vi "Replacing The Heart - Lesson 8.vi"() -> ()   [LabVIEW 2023]
doc: "This lesson uses malleable VIs and LabVIEW classes without dynamic dispatching to solve the problem. The lesson introduces the concept of using malleable VIs to define an interface then allowing multiple LabVIEW classes to implement that interface."
uses:
  Person Information.ctl
  People Wrapper/People Wrapper.lvclass
  People Wrapper/People Wrapper.lvclass/People Wrapper.ctl
  791c92dc-b78f-4473-b048-a19d6874acda.vi
  45d1eefa-c392-4e6e-b1eb-d27fc55e6400.vi
  b0cddedf-f79d-4358-86cb-e9457ff97cbf.vi
  People Wrapper/Write Person.vi
  People Wrapper/Read Person.vi
  People Wrapper/Less Than.vi
  People By Year Wrapper/People By Year Wrapper.lvclass
  People By Name Wrapper/People By Name Wrapper.lvclass
panel:
  in  "Sort By":string(combo)="Default"
  in  "Stop":bool
  out "Sorted People":T1[](array[typedef]) {"Birth Date" format="%<%Y/%b/%d>T"}
  in  "Unsorted People":T1[](array[typedef])=[{"ID"=0, "Family Name"="Tennant", "Given Name"="David", "Birth Date"=timestamp(-6434737636.184167 s since 1904-01-01)}, {"ID"=1, "Family Name"="Smith", "Given Name"="Matt", "Birth Date"=timestamp(-6434726400 s since 1904-01-01)}, {"ID"=2, "Family Name"="Li", "Given Name"="Jing", "Birth Date"=timestamp(3091380833.9038334 s since 1904-01-01)}, {"ID"=3, "Family Name"="Patel", "Given Name"="Aadhya", "Birth Date"=timestamp(3093541462.901833 s since 1904-01-01)}, {"ID"=4, "Family Name"="Doe", "Given Name"="Jane", "Birth Date"=timestamp(3154453586.3918333 s since 1904-01-01)}, {"ID"=5, "Family Name"="Rahman", "Given Name"="Mohammed", "Birth Date"=timestamp(3024418078.500833 s since 1904-01-01)}] {"Birth Date" format="%<%Y/%b/%d>T"}
  # "Overview: This lesson is a fourth way to replace core functions. As with the previous three techniques, this lesson starts with the simple case of wanting to replace the function at the heart of an algorithm, without needing parameterization. This time, we will use malleable VIs to create interfaces that LabVIEW classes can fulfill.\n\nIf you are unfamiliar with malleable VIs, you likely want to review other examples first: \n  *  Malleable VIs\\Basics\n  *  Malleable VIs\\Class Adaptation\n\nInstructions:\n1. Run the VI. The data will be sorted. In this lesson, you cannot choose different sort orders.\n2. Look at the block diagram to see how the sort is done.\n3. Proceed to the next lesson."
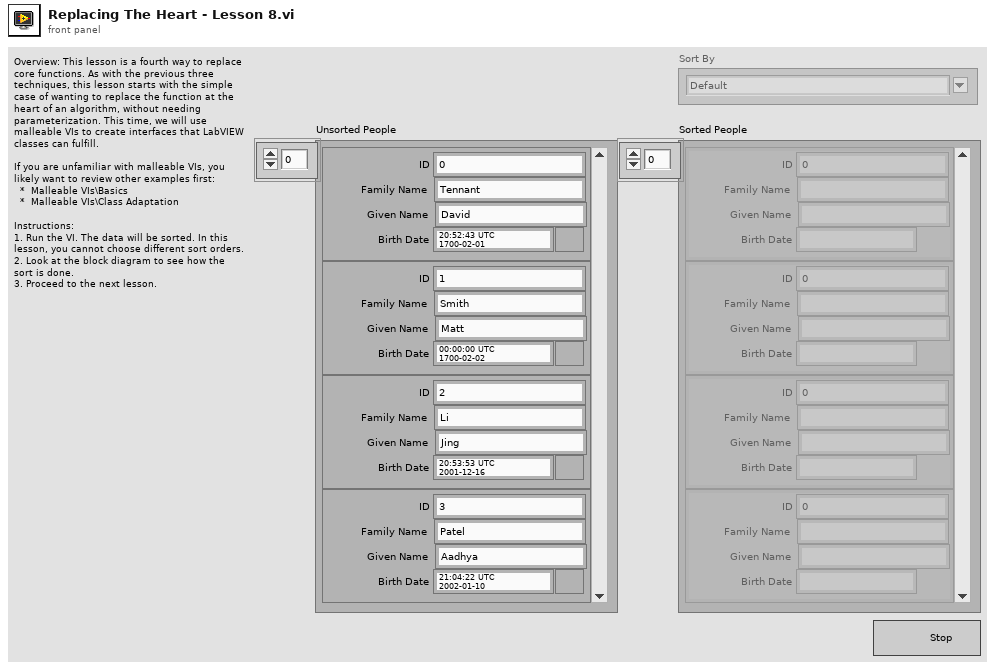
[diagram p1: front panel]
types:
  T1 = typedef "Person Information.ctl" = cluster{"ID":u32, "Family Name":string, "Given Name":string, "Birth Date":timestamp}
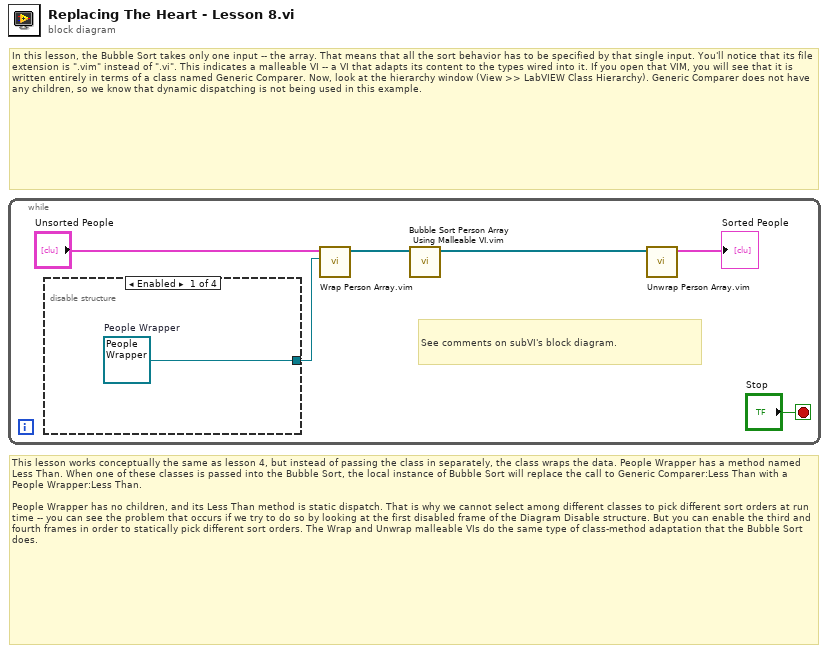
[diagram p0: block diagram]
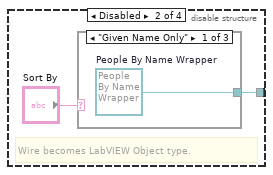
[diagram p2: hidden frame]
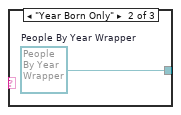
[diagram p3: hidden frame]
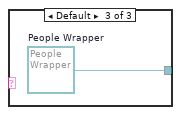
[diagram p4: hidden frame]
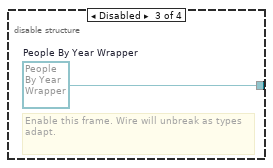
[diagram p5: hidden frame]
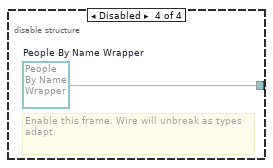
[diagram p6: hidden frame]
diagram:
  # "This lesson works conceptually the same as lesson 4, but instead of passing the class in separately, the class wraps the data. People Wrapper has a method named Less Than. When one of these classes is passed into the Bubble Sort, the local instance of Bubble Sort will replace the call to Generic Comparer:Less Than with a People Wrapper:Less Than.\n\nPeople Wrapper has no children, and its Less Than method is static dispatch. That is why we cannot select among different classes to pick different sort orders at run time -- you can see the problem that occurs if we try to do so by looking at the first disabled frame of the Diagram Disable structure. But you can enable the third and fourth frames in order to statically pick different sort orders. The Wrap and Unwrap malleable VIs do the same type of class-method adaptation that the Bubble Sort does."
  # "In this lesson, the Bubble Sort takes only one input -- the array. That means that all the sort behavior has to be specified by that single input. You'll notice that its file extension is \".vim\" instead of \".vi\". This indicates a malleable VI -- a VI that adapts its content to the types wired into it. If you open that VIM, you will see that it is written entirely in terms of a class named Generic Comparer. Now, look at the hierarchy window (View >> LabVIEW Class Hierarchy). Generic Comparer does not have any children, so we know that dynamic dispatching is not being used in this example."
  n1 = while {
    stop <- "Stop" stop-if-true
    # "See comments on subVI's block diagram."
    n2 = disable-structure shown="Enabled" {
      disable-tunnel: [w7 w8 w13 w14] -> w1
      frame Enabled {
        w7 = refnum<class "People Wrapper.lvclass"> refnum  # People Wrapper
      }
      frame Disabled {
        # "Wire becomes LabVIEW Object type."
        n3 = case shown="\"Given Name Only\"" "Sort By" {
          tunnel: [w10 w11 w12] -> w8
          frame "Given Name Only" {
            w10 = refnum<class "People By Name Wrapper.lvclass"> refnum  # People By Name Wrapper
          }
          frame "Year Born Only" {
            w11 = refnum<class "People By Year Wrapper.lvclass"> refnum  # People By Year Wrapper
          }
          frame Default {
            w12 = refnum<class "People Wrapper.lvclass"> refnum  # People Wrapper
          }
        }
      }
      frame Disabled {
        w13 = refnum<class "People By Year Wrapper.lvclass"> refnum  # People By Year Wrapper
        # "Enable this frame. Wire will unbreak as types adapt."
      }
      frame Disabled {
        w14 = refnum<class "People By Name Wrapper.lvclass"> refnum  # People By Name Wrapper
        # "Enable this frame. Wire will unbreak as types adapt."
      }
    }
    n4 = call "Wrap Person Array.vim"("People Wrapper in"=w1, "Unsorted People"="Unsorted People") -> ("Array"=w5:refnum<class "People Wrapper.lvclass">[])  [unwired: 9 in]
    n5 = call "Bubble Sort Person Array Using Malleable VI.vim"("Unsorted"=w5) -> ("Sorted"=w3:refnum<class "People Wrapper.lvclass">[])  [unwired: 10 in]
    n6 = call "Unwrap Person Array.vim"("Sorted"=w3) -> ("Array"=→"Sorted People":T1[])  [unwired: 10 in]
  }
